vi "step_motor.vi"(6 "F_Threshold":fxp<+,12,12>, 8 "dtau_mr":fxp<+,64,32>, 10 "omega_y":fxp<+/-,20,9>, 11 "F":fxp<+/-,20,10>) -> (1 "vq_F":fxp<+/-,20,5> format="%.57g", 3 "vd_F":fxp<+/-,20,5>)   [LabVIEW 2014]
uses:
  <vilib>/rvi/FXPMathLib/FxpMul/XNode/nifxpmath_Multiplier.xnode
  <vilib>/rvi/FXPMathLib/FxpAdd/XNode/nifxpmath_Add.xnode
  <vilib>/rvi/FXPMathLib/sim/FxpSim.dll
panel:
  out "Lmdtau_mr/Km":fxp<+/-,30,15>
  out "-RKm/NrL":fxp<+/-,18,3>=-1.9615478515625
  out "tauR/Km":fxp<+/-,30,15>
  out "Kmw":fxp<+/-,25,10> format="%.50g"
  out "-NrLwtau/Km":fxp<+/-,36,21> format="%.54g"
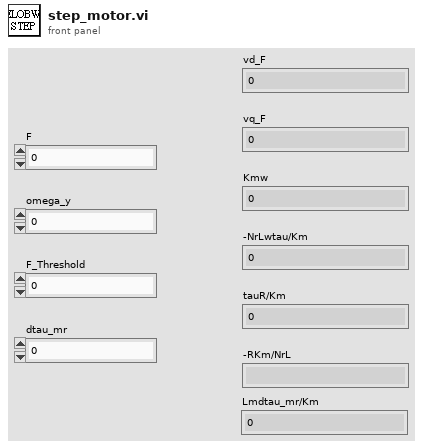
[diagram p1: front panel]
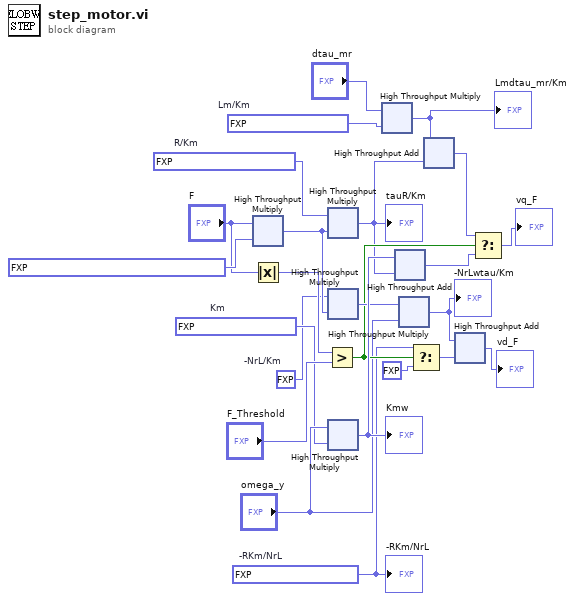
[diagram p0: block diagram]
diagram:
  w2 = fxp<+,23,7> 0.191741943359375  # Lm/Km
  w6 = fxp<+/-,20,4> -8.0  # -NrL/Km
  w7 = fxp<+/-,18,3> -0.943389892578125  # -RKm/NrL
  w8 = fxp<+,23,7> 106.75270080566406  # R/Km
  w9 = fxp<+,14,-2> 0.092193603515625  # Km
  n1 = xnode ("High Throughput Multiply")("x"="F", "y"=fxp<+/-,28,0> -0.0003853030502796173) -> ("x*y"=w21:fxp<+/-,15,-1>)
  n2 = Absolute Value(x="F") -> (abs(x)=w20:fxp<+,20,10>)
  n3 = Greater?(x=w20, y="F_Threshold") -> (0:w14:bool)
  n4 = xnode ("High Throughput Multiply")("x"=w8, "y"=w21) -> ("x*y"=w5:fxp<+/-,20,5>)
  "tauR/Km" <- w5
  n5 = xnode ("High Throughput Multiply")("x"=w6, "y"=w21) -> ("x*y"=w23:fxp<+/-,17,1>)
  n6 = xnode ("High Throughput Multiply")("x"="omega_y", "y"=w9) -> ("x*y"=w24:fxp<+/-,22,7>)
  "Kmw" <- w24
  n7 = xnode ("High Throughput Multiply")("x"="dtau_mr", "y"=w2) -> ("x*y"=w1:fxp<+/-,20,5>)
  "Lmdtau_mr/Km" <- w1
  n8 = xnode ("High Throughput Add")("x"=w24, "y"=w5) -> ("x+y"=w13:fxp<+/-,20,5>)
  n9 = xnode ("High Throughput Multiply")("x"=w23, "y"="omega_y") -> ("x*y"=w18:fxp<+/-,20,5>)
  "-NrLwtau/Km" <- w18
  n10 = Select(t=w7, s=w14, f=fxp<+/-,18,3> 0.0) -> (s? t:f=w16:fxp<+/-,18,3>)
  n11 = xnode ("High Throughput Add")("x"=w1, "y"=w5) -> ("x+y"=w4:fxp<+/-,20,5>)
  n12 = xnode ("High Throughput Add")("x"=w18, "y"=w16) -> ("x+y"=→"vd_F":fxp<+/-,20,5>)
  n13 = Select(t=w4, s=w14, f=w13) -> (s? t:f=→"vq_F":fxp<+/-,20,5>)
  "-RKm/NrL" <- w7
